vi "GetState.vi"(8 "error in (no error)":errorcluster, 11 "reference in":refnum<class "Switch_Keysight_34934A.lvclass">) -> (0 "error out":errorcluster, 1 "States":bool[](array[boolean]), 2 "Routes":string[](array[string]), 3 "reference in":refnum<class "Switch_Keysight_34934A.lvclass">)   [LabVIEW 2022 SP3, in "Switch_Keysight_34934A.lvlib" / "Switch_Keysight_34934A.lvclass"]
uses:
  Switch_Keysight_34934A.lvclass
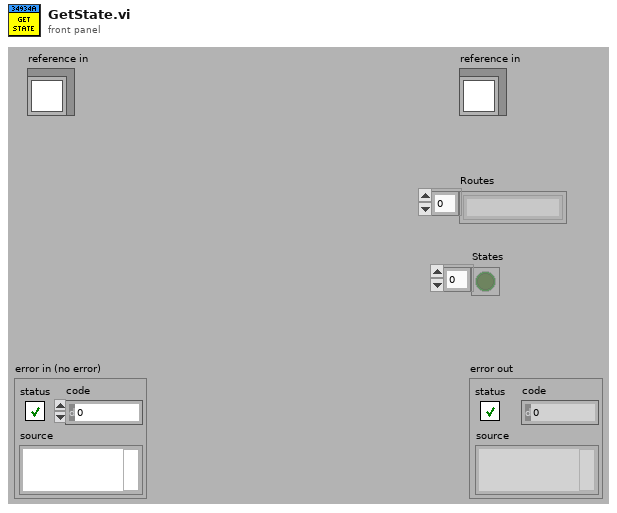
[diagram p1: front panel]
types:
  T1 = typedef "Switch_Keysight_34934A.lvlib/Switch_Keysight_34934A.lvclass/ObjectAttributes.ctl" = cluster{"Config":T2, "VISA ref":refnum<visa-resource-name>, "M1H":bool[][], "M2H":bool[][], "M1L":bool[][], "M2L":bool[][], "route":string, "State":bool[], "StateModBit":bool[], "UpdateEvent":refnum<user-event>}
  T2 = typedef "Switch_Keysight_34934A.lvlib/Switch_Keysight_34934A.lvclass/Config.ctl" = cluster{"VISA":refnum<visa-resource-name>, "Slot":i32, "SwitchMap":cluster{"Name":string, "Route":string[], "UnRoute":string[], "Description":string, "Group":string, "IsGroup":bool}[], "Sim":bool}
  T3 = cluster{"Name":string, "Route":string[], "UnRoute":string[], "Description":string, "Group":string, "IsGroup":bool}[]
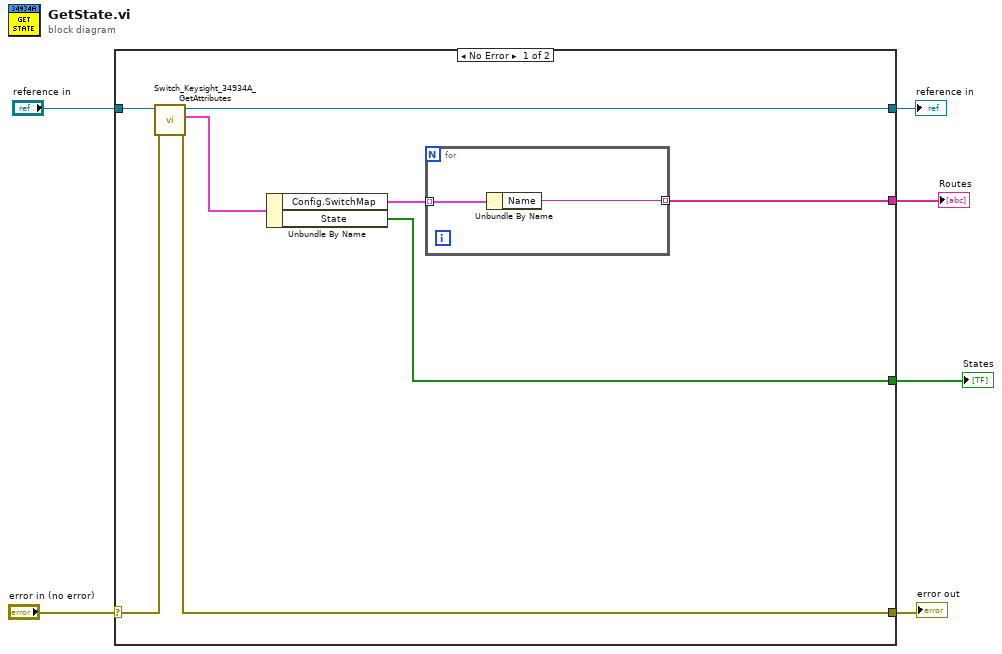
[diagram p0: block diagram]
diagram:
  n1 = case shown="No Error" "error in (no error)" {
    selector: "error in (no error)" -> [w14 w18]
    tunnel: [w12 w18] -> w5
    tunnel: [w10 w17] -> w3
    tunnel: "reference in" -> [w11 w17]
    tunnel: [w8 _] -> w2
    tunnel: [w7 _] -> w1
    frame No Error {
      n2 = call "Switch_Keysight_34934A_GetAttributes.vi"("error in (no error)"=w14, "reference in"=w11) -> ("error out"=w12:errorcluster, "Data"=w13:T1, "reference out"=w10:refnum<class "Switch_Keysight_34934A.lvclass">)  [unwired: 6 in, 1 out]
      n3 = Unbundle By Name(w13) -> ("Config.SwitchMap"=w9:T3, "State"=w7:bool[])
      n4 = for {
        tunnel: w9 -> [w16] mode=indexing
        tunnel: [w15] -> w8 mode=indexing
        n5 = Unbundle By Name(w16) -> ("Name"=w15:string)
      }
    }
    frame Error {
    }
  }
  "error out" <- w5
  "reference in" <- w3
  "States" <- w1
  "Routes" <- w2
